vi "classes.vi"(0 "HGF_OMFactory":refnum<class "HGF_OMFactory.lvclass">, 1 "className":string, 5 "error in (no error)":errorcluster) -> (14 "HGF_OMFactory dup":refnum<class "HGF_OMFactory.lvclass">, 16 "Object":refnum<class>, 19 "error out":errorcluster)   [LabVIEW 2012, in "HGF_ObjectManager.lvlib" / "HGF_OMFactory.lvclass"]
doc: "This dynamaic dispatch VI contains constant objects of all classes that can be produced by HGF_Factory.\nClass has to be defined by name. \n\nOptionally, you can also specifiy a Class Path String instead, but you have to make sure that all dependencies are available.\n\nChild classes have to override it to define additional classes."
uses:
  HGF_OMFactory.lvclass
  HGF_BaseClasses/HGF_TaskEventListener/HGF_TaskEventListener.lvclass
  HGF_BaseClasses/HGF_Factory/HGF_Factory.lvclass
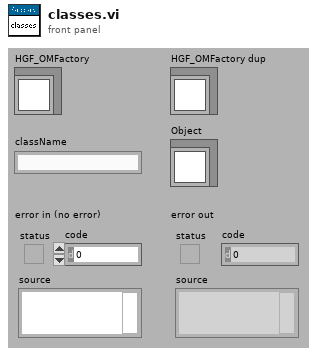
[diagram p1: front panel]
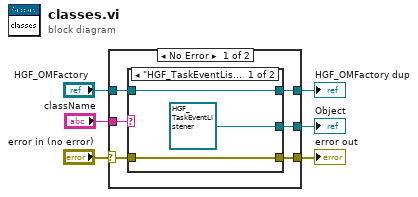
[diagram p0: block diagram]
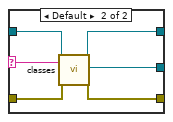
[diagram p2: hidden frame]
diagram:
  n1 = case shown="No Error" "error in (no error)" {
    selector: "error in (no error)" -> [w7 w22]
    tunnel: "HGF_OMFactory" -> [w12 w23]
    tunnel: [w11 w23] -> w5
    tunnel: [w10 _] -> w4
    tunnel: [w9 w22] -> w3
    tunnel: "className" -> [w8 _]
    frame No Error {
      n2 = case shown="\"HGF_TaskEventListener\"" w8 {
        selector: w8 -> [_ w16]
        tunnel: w12 -> [w14 w21]
        tunnel: w7 -> [w13 w20]
        tunnel: [w14 w19] -> w11
        tunnel: [refnum<class "HGF_TaskEventListener.lvclass"> refnum ("HGF_BaseClasses.lvlib:HGF_TaskEventListener.lvclass") w18] -> w10
        tunnel: [w13 w17] -> w9
        frame "HGF_TaskEventListener" {
        }
        frame Default {
          n3 = call-parent "classes.vi"("HGF_Factory"=w21, "className"=w16, "error in (no error)"=w20) -> ("HGF_Factory dup"=w19:refnum<class "HGF_OMFactory.lvclass">, "Object"=w18:refnum<class>, "error out"=w17:errorcluster)  [unwired: 14 in]
        }
      }
    }
    frame Error {
    }
  }
  "error out" <- w3
  "HGF_OMFactory dup" <- w5
  "Object" <- w4
